vi "Area Scoring Rectangle.vi"(10 "Convex Hull Area":dbl, 11 "Area":dbl) -> (3 "Score":dbl)   [LabVIEW 2019]
doc: "Calculate a score based on area and convex hull area. Convex hull area fills holes and convex areas of the shape. It is equivalent to putting a rubber band around the shape and computing the area enclosed by the band."
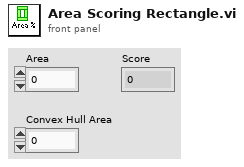
[diagram p1: front panel]
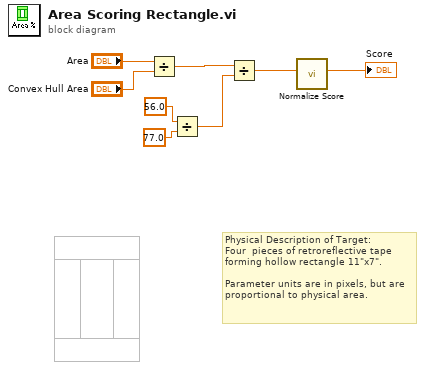
[diagram p0: block diagram]
diagram:
  # "Physical Description of Target:\nFour  pieces of retroreflective tape\nforming hollow rectangle 11\"x7\".\n\nParameter units are in pixels, but are\nproportional to physical area."
  n1 = Divide(x="Area", y="Convex Hull Area") -> (x/y=w7:dbl)
  n2 = Divide(x=56.0 ("length"), y=77.0 ("length")) -> (x/y=w3:dbl)
  n3 = Divide(x=w7, y=w3) -> (x/y=w5:dbl)
  n4 = call "Normalize Score.vi"("Value"=w5) -> ("Score"=→"Score":dbl)  [unwired: 10 in]
